vi "Xeryon convert stage type.vi"(4 "Stage type in":string) -> (1 "Stage type out":string)   [LabVIEW 2019]
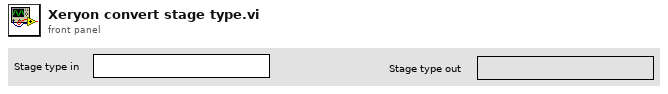
[diagram p1: front panel]
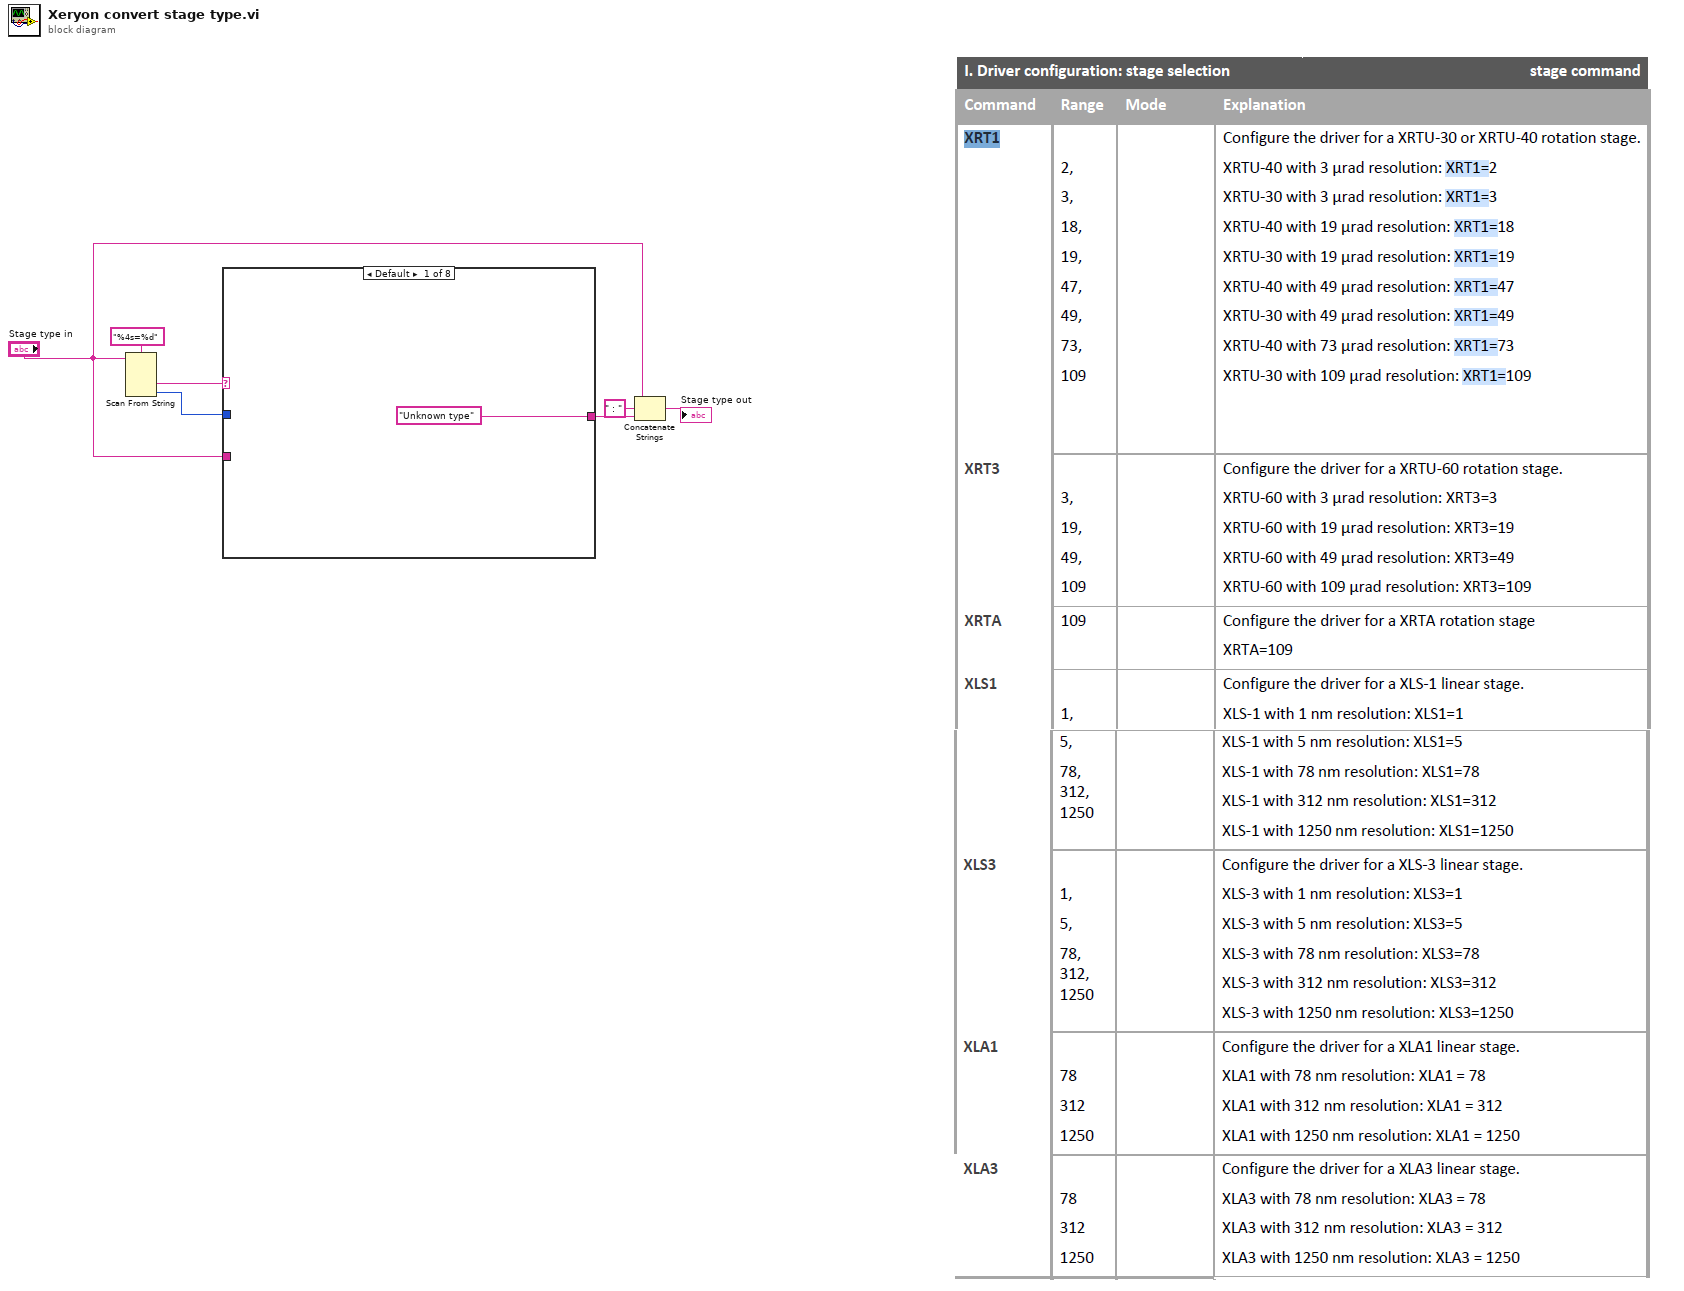
[diagram p0: block diagram]
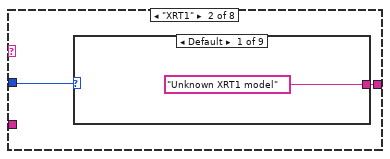
[diagram p2: hidden frame]
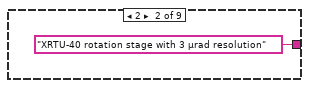
[diagram p3: hidden frame]
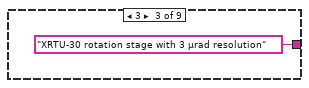
[diagram p4: hidden frame]
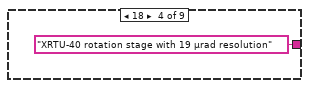
[diagram p5: hidden frame]
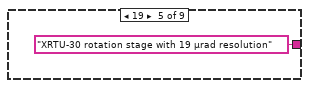
[diagram p6: hidden frame]
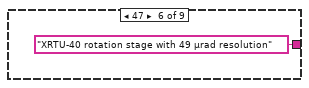
[diagram p7: hidden frame]
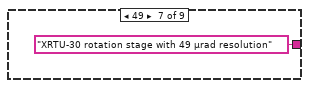
[diagram p8: hidden frame]
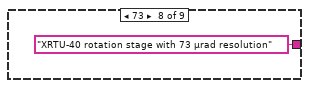
[diagram p9: hidden frame]
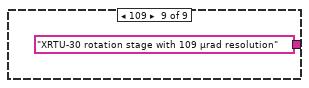
[diagram p10: hidden frame]
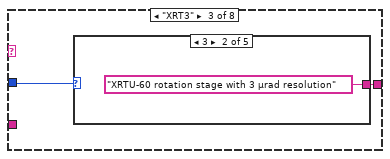
[diagram p11: hidden frame]
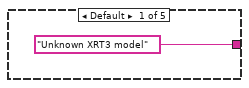
[diagram p12: hidden frame]
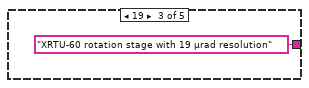
[diagram p13: hidden frame]
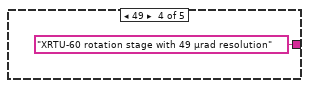
[diagram p14: hidden frame]
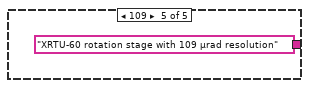
[diagram p15: hidden frame]
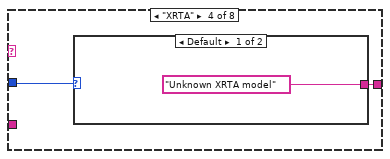
[diagram p16: hidden frame]
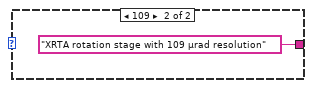
[diagram p17: hidden frame]
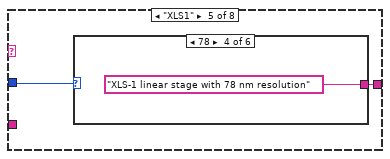
[diagram p18: hidden frame]
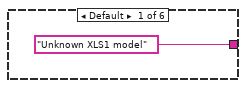
[diagram p19: hidden frame]
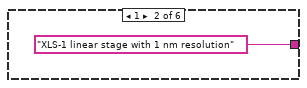
[diagram p20: hidden frame]
diagram:
  n1 = Scan From String(format string="%4s=%d", input string="Stage type in") -> (output 1=w6:string, output 2=w5:i32)  [unwired: 4 in, 3 out]
  n2 = case shown="Default" w6 {
    tunnel: w5 -> [_ w10 w21 w28 w32 w40 w48 w54]
    tunnel: ["Unknown type" w9 w20 w27 w31 w39 w47 w53] -> w2
    tunnel: "Stage type in" -> [_ _ _ _ _ _ _ _]
    frame Default {
    }
    frame "XRT1" {
      n3 = case shown="Default" w10 {
        tunnel: ["Unknown XRT1 model" "XRTU-40 rotation stage with 3 µrad resolution" "XRTU-30 rotation stage with 3 µrad resolution" "XRTU-40 rotation stage with 19 µrad resolution" "XRTU-30 rotation stage with 19 µrad resolution" "XRTU-40 rotation stage with 49 µrad resolution" "XRTU-30 rotation stage with 49 µrad resolution" "XRTU-40 rotation stage with 73 µrad resolution" "XRTU-30 rotation stage with 109 µrad resolution"] -> w9
        frame Default {
        }
        frame 2 {
        }
        frame 3 {
        }
        frame 18 {
        }
        frame 19 {
        }
        frame 47 {
        }
        frame 49 {
        }
        frame 73 {
        }
        frame 109 {
        }
      }
    }
    frame "XRT3" {
      n4 = case shown="3" w21 {
        tunnel: ["Unknown XRT3 model" "XRTU-60 rotation stage with 3 µrad resolution" "XRTU-60 rotation stage with 19 µrad resolution" "XRTU-60 rotation stage with 49 µrad resolution" "XRTU-60 rotation stage with 109 µrad resolution"] -> w20
        frame Default {
        }
        frame 3 {
        }
        frame 19 {
        }
        frame 49 {
        }
        frame 109 {
        }
      }
    }
    frame "XRTA" {
      n5 = case shown="Default" w28 {
        tunnel: ["Unknown XRTA model" "XRTA rotation stage with 109 µrad resolution"] -> w27
        frame Default {
        }
        frame 109 {
        }
      }
    }
    frame "XLS1" {
      n6 = case shown="78" w32 {
        tunnel: ["Unknown XLS1 model" "XLS-1 linear stage with 1 nm resolution" "XLS-1 linear stage with 5 nm resolution" "XLS-1 linear stage with 78 nm resolution" "XLS-1 linear stage with 312 nm resolution" "XLS-1 linear stage with 1250 nm resolution"] -> w31
        frame Default {
        }
        frame 1 {
        }
        frame 5 {
        }
        frame 78 {
        }
        frame 312 {
        }
        frame 1250 {
        }
      }
    }
    frame "XLS3" {
      n7 = case shown="1250" w40 {
        tunnel: ["Unknown XLS3 model" "XLS-3 linear stage with 1 nm resolution" "XLS-3 linear stage with 5 nm resolution" "XLS-3 linear stage with 78 nm resolution" "XLS-3 linear stage with 312 nm resolution" "XLS-3 linear stage with 1250 nm resolution"] -> w39
        frame Default {
        }
        frame 1 {
        }
        frame 5 {
        }
        frame 78 {
        }
        frame 312 {
        }
        frame 1250 {
        }
      }
    }
    frame "XLA1" {
      n8 = case shown="1250" w48 {
        tunnel: ["Unknown XLA1 model" "XLA1 linear stage with 78 nm resolution" "XLA1linear stage with 312 nm resolution" "XLA1 linear stage with 1250 nm resolution"] -> w47
        frame Default {
        }
        frame 78 {
        }
        frame 312 {
        }
        frame 1250 {
        }
      }
    }
    frame "XLA3" {
      n9 = case shown="1250" w54 {
        tunnel: ["Unknown XLA3 model" "XLA3 linear stage with 78 nm resolution" "XLA3 linear stage with 312 nm resolution" "XLA3 linear stage with 1250 nm resolution"] -> w53
        frame Default {
        }
        frame 78 {
        }
        frame 312 {
        }
        frame 1250 {
        }
      }
    }
  }
  n10 = Concatenate Strings("Stage type in", " : " ("string"), w2) -> (→"Stage type out":string)
